vi "AddEnumToProject.vi"(8 "error in (no error)":errorcluster, 11 "baseClass in":refnum<class "baseClass.lvclass">) -> (0 "error out":errorcluster, 3 "baseClass out":refnum<class "baseClass.lvclass">)   [LabVIEW 2013, in "baseClass.lvclass"]
uses:
  baseClass.lvclass
  ProjectHandler/RefNums.vi
  ProjectHandler.lvlib
  GenLVOOP/GenLVOOP.lvclass
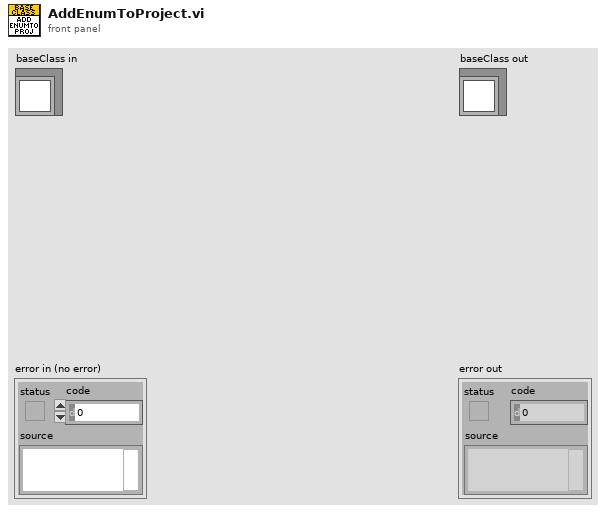
[diagram p1: front panel]
types:
  T1 = cluster{"App":refnum<vi>, "Project":refnum<vi>, "My Computer":refnum<vi>}
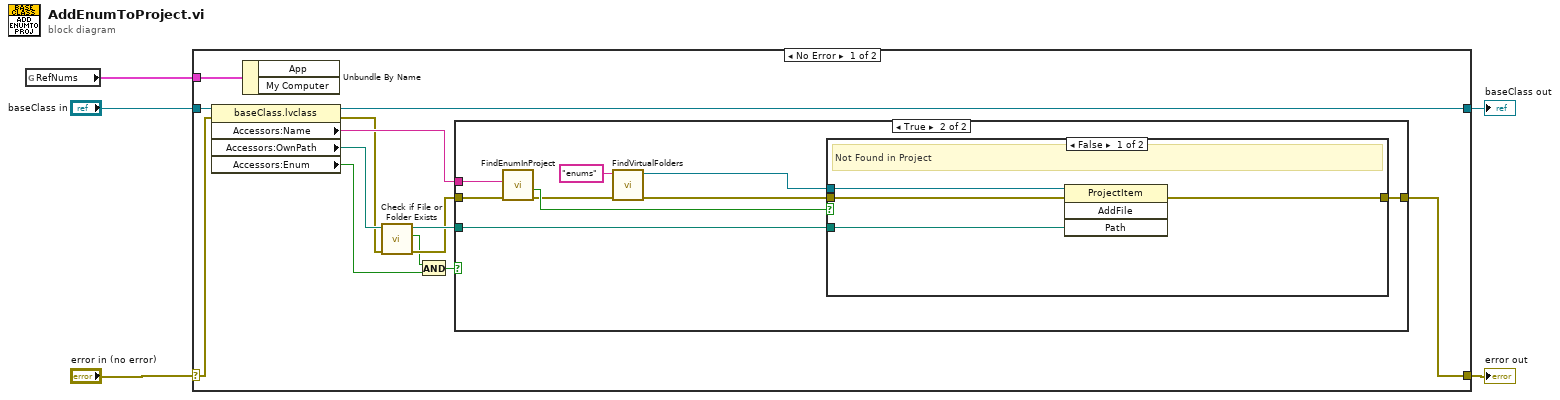
[diagram p0: block diagram]
diagram:
  n1 = global read "RefNums.vi" "RefNums"() -> (w1:T1)
  n2 = case shown="No Error" "error in (no error)" {
    selector: "error in (no error)" -> [w10 w35]
    tunnel: [w9 w35] -> w4
    tunnel: [w17 w34] -> w2
    tunnel: "baseClass in" -> [w18 w34]
    tunnel: w1 -> [w16 _]
    frame No Error {
      n3 = property class="baseClass.lvclass"(reference=w18, error in=w10) -> (reference out=w17:refnum<class "baseClass.lvclass">, error out=w12:errorcluster, "Accessors:Name"=w13:string, "Accessors:OwnPath"=w15:path, "Accessors:Enum"=w8:bool)
      n4 = Unbundle By Name(w16) -> ()  [unwired: 2 out]
      n5 = call <vilib>:"Check if File or Folder Exists.vi"("error in (no error)"=w12, "path"=w15) -> ("error out"=w11:errorcluster, "file or folder exists?"=w7:bool, "dup path"=w14:path)  [unwired: 7 in]
      n6 = And(x=w7, y=w8) -> (x .and. y?=w6:bool)
      n7 = case shown="True" w6 {
        tunnel: w14 -> [_ w27]
        tunnel: w13 -> [_ w24]
        tunnel: w11 -> [w19 w23]
        tunnel: [w19 w28] -> w9
        frame False {
        }
        frame True {
          n8 = call "FindEnumInProject.vi"("error in (no error)"=w23, "Name"=w24) -> ("error out"=w25:errorcluster, "Found"=w26:bool)  [unwired: 7 in, 1 out]
          n9 = call "FindVirtualFolders.vi"("error in (no error)"=w25, "Name"="enums") -> ("error out"=w22:errorcluster, "Folder"=w20:refnum<vi>)  [unwired: 7 in, 1 out]
          n10 = case shown="False" w26 {
            tunnel: w20 -> [w32 _]
            tunnel: w27 -> [w30 _]
            tunnel: w22 -> [w29 w33]
            tunnel: [w31 w33] -> w28
            frame False {
              # "Not Found in Project"
              n11 = invoke class="ProjectItem" method="AddFile"(reference=w32, error in=w29, "Path"=w30) -> (error out=w31:errorcluster)  [unwired: 1 in, 3 out]
            }
            frame True {
            }
          }
        }
      }
    }
    frame Error {
    }
  }
  "error out" <- w4
  "baseClass out" <- w2
